vi "Main.vi"(7 "ConcreteActor":refnum<class "ConcreteActor.lvclass">, 10 "ErrorQueue":refnum<queue>, 11 "PreSetupQueue":refnum<queue>) -> (4 "Error":errorcluster, 5 "ConcreteActor":refnum<class "ConcreteActor.lvclass">)   [LabVIEW 2020, in "jettl.lvlib" / "Base.lvlib" / "ConcreteActor.lvclass"]
uses:
  ConcreteActor.lvclass
  ConcreteActor.lvclass/ConcreteActor.ctl
  PreSetup.ctl
  jettl.lvlib
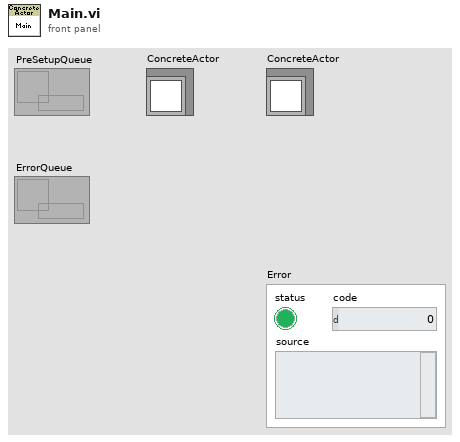
[diagram p1: front panel]
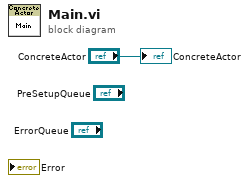
[diagram p0: block diagram]
diagram:
  "ConcreteActor" <- "ConcreteActor"
